vi "Vi Read.vi"(8 "error in (no error)":errorcluster {"code" format="%.0x"}, 9 "BufferSize":i64=2048, 11 "instrument handle":refnum<k15>) -> (0 "error out":errorcluster {"code" format="%.0x"}, 1 "ReturnCount":i64, 2 "Buffer":u32, 3 "instrument handle out":refnum<k15>)   [LabVIEW 2021, in "Keysight XSAnVMA.lvlib"]
doc: "Reads a complete response from the instrument and returns it as an array of bytes."
uses:
  <instrlib>/Keysight XSAnVMA/Keysight XSAnVMA.lvlib
  KtXSAnVMA_64.dll
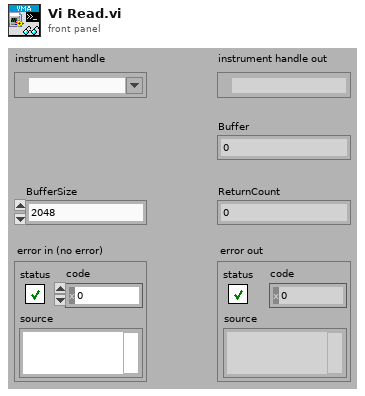
[diagram p1: front panel]
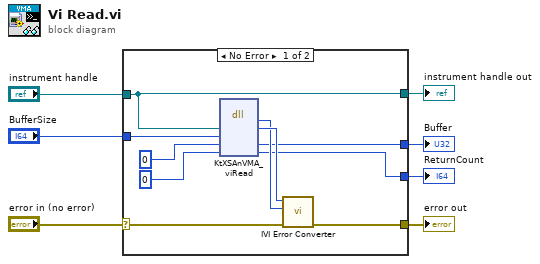
[diagram p0: block diagram]
diagram:
  n1 = case shown="No Error" "error in (no error)" {
    selector: "error in (no error)" -> [w15 w19]
    tunnel: [w14 w19] -> w7
    tunnel: "instrument handle" -> [w8 w18]
    tunnel: "BufferSize" -> [w13 _]
    tunnel: [w11 _] -> w3
    tunnel: [w9 _] -> w2
    tunnel: [w8 w18] -> w1
    frame No Error {
      n2 = dll-call lib="KtXSAnVMA**.dll" fn="KtXSAnVMA_viRead"("Vi"=w8, "BufferSize"=w13, "Buffer"=u32 0, "ReturnCount"=i64 0) -> (w16:i32, "Vi"=w17:u32, "Buffer"=w11:u32, "ReturnCount"=w9:i64)  [unwired: 4 in, 2 out]
      n3 = call <instrlib>:"IVI Error Converter.vi"("error in (no error)"=w15, "IVI error code (0)"=w16, "instrument handle"=w17) -> ("error out"=w14:errorcluster)  [unwired: 7 in, 1 out]
    }
    frame Error {
    }
  }
  "error out" <- w7
  "instrument handle out" <- w1
  "Buffer" <- w3
  "ReturnCount" <- w2
